vi "test_EmptyInstrumentTypeId_CallCreateSessions_ReturnsError.vi"(8 "error in":errorcluster) -> (0 "error out":errorcluster, 2 "result":string, 3 "pass":bool)   [LabVIEW 2020, in "MeasurementServerTests.lvlib"]
uses:
  MeasurementServerTests.lvlib
  da6ffb6f-c1c9-4957-84dd-e9228483c454.vi
  Helpers/Fake Instrument/Fake Instrument.lvclass
  \\tsclient\C/dev/measurementlink-labview/Source/Runtime/MeasurementLink Instrument/IInstrument/IInstrument.lvclass
  Runtime/MeasurementLink Measurement Server/Helpers/Error Strings Global Internal.vi
  Runtime/MeasurementLink Session Management/Session Reservation/Create Sessions Impl.vi
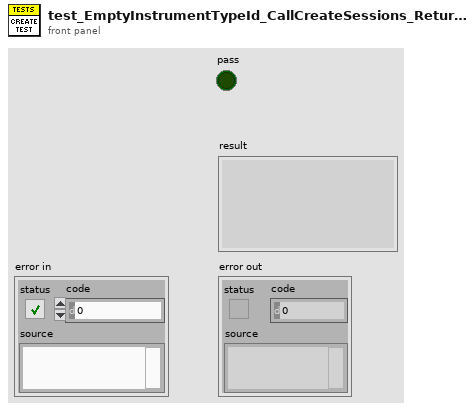
[diagram p1: front panel]
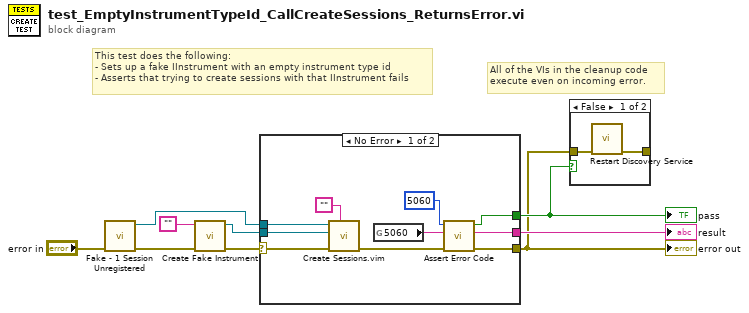
[diagram p0: block diagram]
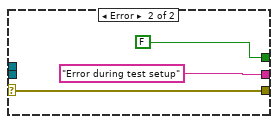
[diagram p2: hidden frame]
diagram:
  # "All of the VIs in the cleanup code\nexecute even on incoming error."
  # "This test does the following:\n- Sets up a fake IInstrument with an empty instrument type id\n- Asserts that trying to create sessions with that IInstrument fails"
  n1 = call "Fake - 1 Session Unregistered.vi"("error in"="error in") -> ("error out"=w6:errorcluster, "session reservation out"=w2:refnum<class "Session Reservation.lvclass">)  [unwired: 9 in]
  n2 = call "Create Fake Instrument.vi"("error in"=w6, "instrument type id"="") -> ("error out"=w4:errorcluster, "fake instrument out"=w3:refnum<class "Fake Instrument.lvclass">)  [unwired: 8 in]
  n3 = case shown="No Error" w4 {
    selector: w4 -> [w17 w20]
    tunnel: [w15 w20] -> w7
    tunnel: [w14 FALSE] -> w8
    tunnel: [w13 "Error during test setup" ("f")] -> w9
    tunnel: w3 -> [w19 _]
    tunnel: w2 -> [w18 _]
    frame No Error {
      n4 = call "Create Sessions.vim"("session type"="", "error in"=w17, "instrument"=w19, "session reservation in"=w18) -> ("error out"=w16:errorcluster)  [unwired: 4 in, 3 out]
      n5 = global read "Error Strings Global Internal.vi" "5060"() -> (w10:string)
      n6 = call "Assert Error Code.vi"("error in"=w16, "expected error description"=w10, "expected error code"=5060) -> ("error out"=w15:errorcluster, "details"=w13:string, "error code match?"=w14:bool)  [unwired: 6 in]
    }
    frame Error {
    }
  }
  "error out" <- w7
  "pass" <- w8
  "result" <- w9
  n7 = case shown="False" w8 {
    tunnel: w7 -> [w24 _]
    tunnel: [w23 _] -> _
    frame False {
      n8 = call "Restart Discovery Service.vi"("error in"=w24) -> ("error out"=w23:errorcluster)  [unwired: 10 in]
    }
    frame True {
    }
  }
